vi "Switch Convert Stimulus Cluster.vi"(4 "Conversion":enum16{"Cluster - HTML", "HTML - Cluster"}(ring), 6 "Stimulus Key Array In":T7, 7 "Stimulus Cluster In":T5) -> (1 "Stimulus Cluster Out":T5, 2 "Stumulus HTML Out":string)   [LabVIEW 2011]
uses:
  ITK EXT/utils/keyedarr.llb/Keyed Array.ctl
  TypeDefs/Switch Stimulus Parameters.ctl
  TypeDefs/Switch Type.ctl
  drivers/SWI/Kaelus/TypeDefs/Kaelus SWI Position.ctl
  BPIMCore EXT/WebEngine/LIB/MODULES/SW Module/SW Tx Positions.ctl
  BPIMCore EXT/WebEngine/LIB/MODULES/SW Module/SW Rx Positions.ctl
  drivers/PFE/Kaelus/TypeDefs/Kaelus PFE Position.ctl
  ITK EXT/utils/strutil.llb/Case Matching.ctl
panel:
  in  "Switch Position (PFE)":T1
  in  "Switch Position (SWI)":T2
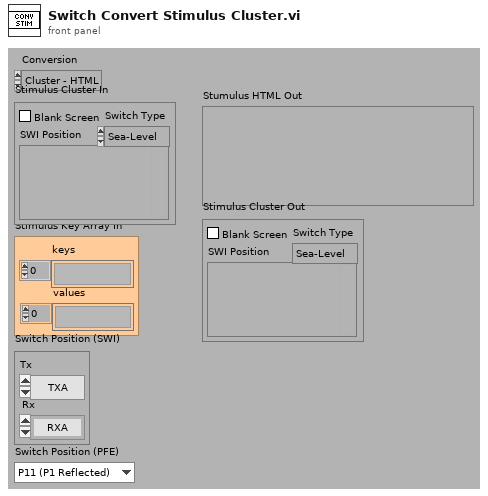
[diagram p1: front panel]
types:
  T1 = typedef "Kaelus PFE Position.ctl" = enum16{"P11 (P1 Reflected)", "P12 (P2 Through)", "P21 (P1 Through)", "P22 (P2 Reflected)"}
  T2 = typedef "Kaelus SWI Position.ctl" = cluster{"Tx":T3, "Rx":T4}
  T3 = typedef "SW Tx Positions.ctl" = enum16{"TXA", "TXB", "TXC"}
  T4 = typedef "SW Rx Positions.ctl" = enum16{"RXA", "RXB", "RXC", "RXD", "RXE", "RXF"}
  T5 = typedef "Switch Stimulus Parameters.ctl" = cluster{"Blank Screen":bool, "SWI Position":variant, "Switch Type":T6}
  T6 = typedef "Switch Type.ctl" = enum16{"Sea-Level", "Simulator", "SI-0206-SW", "SI-0309-SW", "SI-0310-SW", "Front End"}
  T7 = typedef "Keyed Array.ctl" = cluster{"keys":string[], "values":string[]}
  T8 = typedef "Case Matching.ctl" = enum16{"a != A", "a == A", "system"}
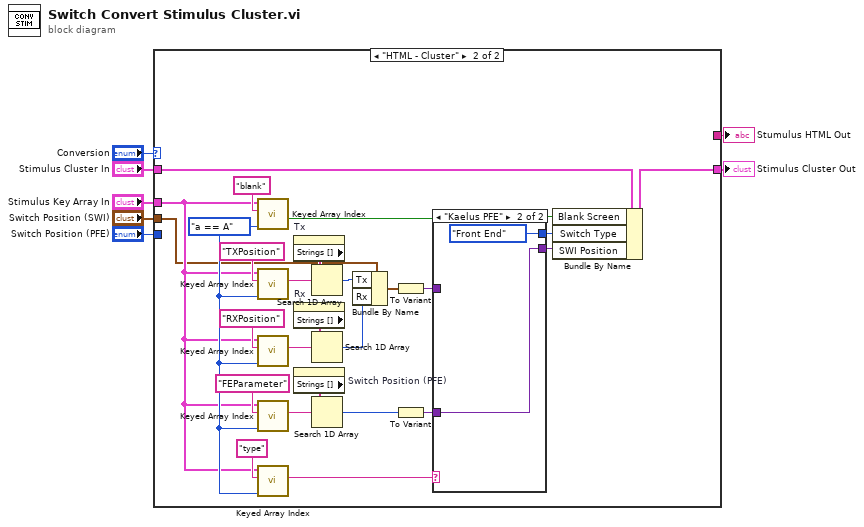
[diagram p0: block diagram]
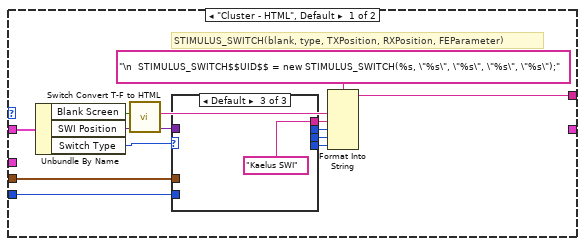
[diagram p2: hidden frame]
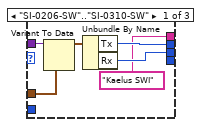
[diagram p3: hidden frame]
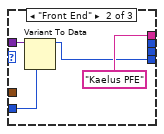
[diagram p4: hidden frame]
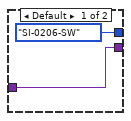
[diagram p5: hidden frame]
diagram:
  n1 = case shown="\"HTML - Cluster\"" "Conversion" {
    tunnel: "Stimulus Cluster In" -> [w20 w57]
    tunnel: "Stimulus Key Array In" -> [_ w39]
    tunnel: [w18 _] -> w4
    tunnel: [_ w56] -> w3
    tunnel: "Switch Position (SWI)" -> [w14 w38]
    tunnel: "Switch Position (PFE)" -> [w12 _]
    frame "Cluster - HTML", Default {
      # "STIMULUS_SWITCH(blank, type, TXPosition, RXPosition, FEParameter)"
      n2 = Unbundle By Name(w20) -> ("Blank Screen"=w17:bool, "SWI Position"=w15:variant, "Switch Type"=w11:T6)
      n3 = call "Switch Convert T-F to HTML.vi"("(T/F)"=w17) -> ("HTML (true/false)"=w16:string)  [unwired: 10 out]
      n4 = case shown="Default" w11 {
        tunnel: w15 -> [w26 w30 _]
        tunnel: w14 -> [w25 _ _]
        tunnel: [w24 _ _] -> w13
        tunnel: w12 -> [_ w28 _]
        tunnel: [w22 _ _] -> w10
        tunnel: ["Kaelus SWI" ("format string") "Kaelus PFE" ("format string") "Kaelus SWI" ("format string")] -> w9
        tunnel: [_ w27 _] -> w8
        frame "SI-0206-SW".."SI-0310-SW" {
          n5 = Variant To Data(type=w25, Variant=w26) -> (data=w23:T2)  [unwired: 1 in, 1 out]
          n6 = Unbundle By Name(w23) -> ("Tx"=w24:T3, "Rx"=w22:T4)
        }
        frame "Front End" {
          n7 = Variant To Data(type=w28, Variant=w30) -> (data=w27:T1)  [unwired: 1 in, 1 out]
        }
        frame Default {
        }
      }
      n8 = Format Into String(format string="\n  STIMULUS_SWITCH$$UID$$ = new STIMULUS_SWITCH(%s, \"%s\", \"%s\", \"%s\", \"%s\");", w16, w9, w13, w10, w8) -> (resulting string=w18:string)  [unwired: 2 in, 1 out]
    }
    frame "HTML - Cluster" {
      w41 = Case_Matching."a == A" ("case matching (sensitive)")
      n9 = call "Keyed Array Index.vi"("case matching (sensitive)"=w41, "key"="blank", "array in"=w39) -> ("valid key"=w53:bool)  [unwired: 1 in, 3 out]
      n10 = call "Keyed Array Index.vi"("case matching (sensitive)"=w41, "key"="TXPosition", "array in"=w39) -> ("value"=w46:string)  [unwired: 1 in, 3 out]
      n11 = call "Keyed Array Index.vi"("case matching (sensitive)"=w41, "key"="RXPosition", "array in"=w39) -> ("value"=w45:string)  [unwired: 1 in, 3 out]
      n12 = call "Keyed Array Index.vi"("case matching (sensitive)"=w41, "key"="FEParameter", "array in"=w39) -> ("value"=w40:string)  [unwired: 1 in, 3 out]
      n13 = call "Keyed Array Index.vi"("case matching (sensitive)"=w41, "key"="type", "array in"=w39) -> ("value"=w37:string)  [unwired: 1 in, 3 out]
      n14 = property on="Tx" class="Enum (strict)"() -> ("Strings []"=w52:string[])  [unwired: 2 in, 2 out]
      n15 = property on="Rx" class="Enum (strict)"() -> ("Strings []"=w50:string[])  [unwired: 2 in, 2 out]
      n16 = property on="Switch Position (PFE)" class="Enum (strict)"() -> ("Strings []"=w44:string[])  [unwired: 2 in, 2 out]
      n17 = Search 1D Array(1D array=w52, element=w46) -> (index of element=w48:i32)  [unwired: 1 out]
      n18 = Search 1D Array(1D array=w50, element=w45) -> (index of element=w49:i32)  [unwired: 1 out]
      n19 = Search 1D Array(1D array=w44, element=w40) -> (index of element=w32:i32)  [unwired: 1 out]
      n20 = Bundle By Name(cluster=w38, "Tx"=w48, "Rx"=w49) -> (w47:T2)
      n21 = To Variant(anything=w47) -> (Variant=w35:variant)
      n22 = To Variant(anything=w32) -> (Variant=w36:variant)
      n23 = case shown="\"Kaelus PFE\"" w37 {
        tunnel: w36 -> [_ w60]
        tunnel: w35 -> [w59 _]
        tunnel: [w59 w60] -> w34
        tunnel: [Switch_Type."SI-0206-SW" ("Switch Type") Switch_Type."Front End" ("Switch Type")] -> w33
        frame Default {
        }
        frame "Kaelus PFE" {
        }
      }
      n24 = Bundle By Name(cluster=w57, "Blank Screen"=w53, "Switch Type"=w33, "SWI Position"=w34) -> (w56:T5)
    }
  }
  "Stumulus HTML Out" <- w4
  "Stimulus Cluster Out" <- w3
